vi "Title No. and Centroid.vi"(2 "半径":dbl, 3 "Particle Measurements (Pixels)":dbl[][](array[numeric])) -> (0 "粒子数":i32, 1 "输出数组":T1(array[cluster]))   [LabVIEW 2016]
panel:
  out "子数组":dbl[](array[numeric])
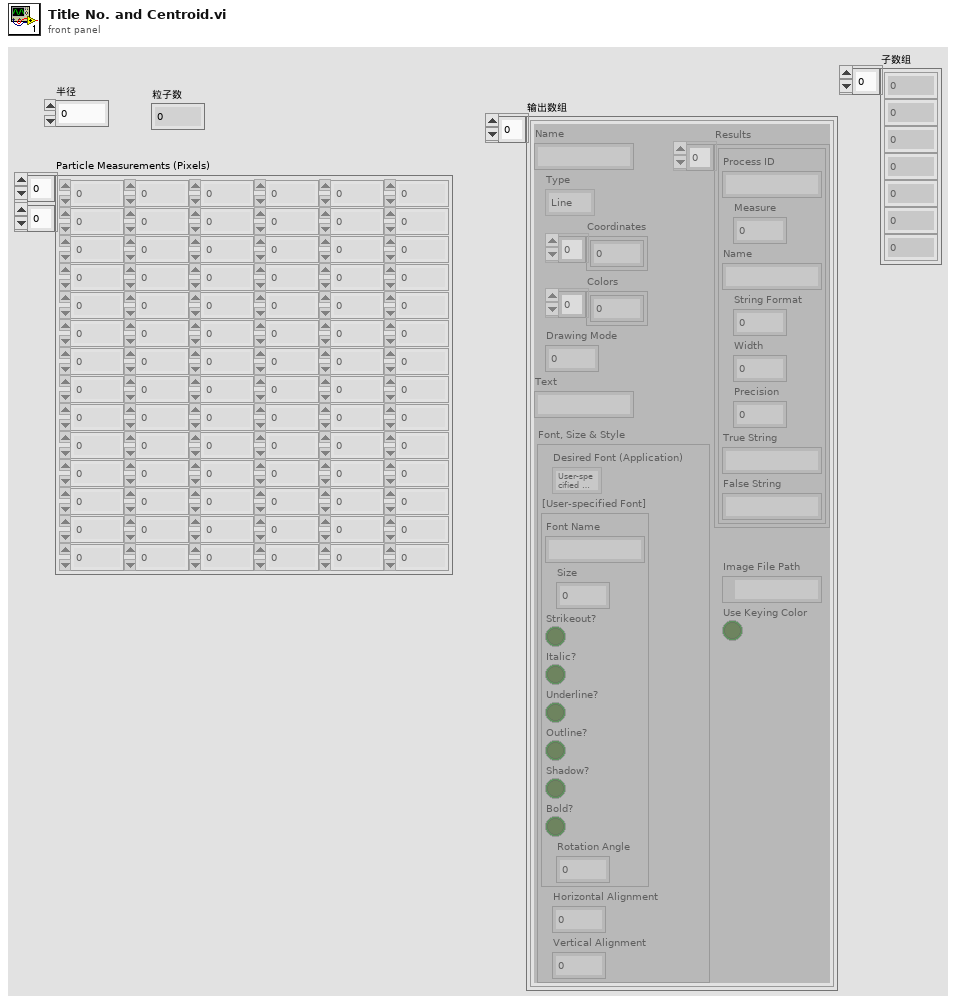
[diagram p1: front panel]
types:
  T1 = cluster{"Name":string, "Type":enum16{"Line", "Broken Line", "Free Hand Line", "Rotated Rectangle", "Oval", "Polygon", "Free Hand", "Bitmap", "Text"}, "Coordinates":i32[], "Colors":u32[], "Drawing Mode":u32, "Text":string, "Results":cluster{"Process ID":string, "Measure":u16, "Name":string, "String Format":u16, "Width":i16, "Precision":i16, "True String":string, "False String":string}[], "Font, Size & Style":cluster{"Desired Font (Application)":enum16{"User-specified Font", "Application Font", "System Font", "Dialog Font"}, "[User-specified Font]":cluster{"Font Name":string, "Size":i16, "Strikeout?":bool, "Italic?":bool, "Underline?":bool, "Outline?":bool, "Shadow?":bool, "Bold?":bool, "Rotation Angle":dbl}, "Horizontal Alignment":i16, "Vertical Alignment":i16}, "Image File Path":path, "Use Keying Color":bool}[]
  T2 = enum16{"Line", "Broken Line", "Free Hand Line", "Rotated Rectangle", "Oval", "Polygon", "Free Hand", "Bitmap", "Text"}
  T3 = cluster{"Name":string, "Type":enum16{"Line", "Broken Line", "Free Hand Line", "Rotated Rectangle", "Oval", "Polygon", "Free Hand", "Bitmap", "Text"}, "Coordinates":i32[], "Colors":u32[], "Drawing Mode":u32, "Text":string, "Results":cluster{"Process ID":string, "Measure":u16, "Name":string, "String Format":u16, "Width":i16, "Precision":i16, "True String":string, "False String":string}[], "Font, Size & Style":cluster{"Desired Font (Application)":enum16{"User-specified Font", "Application Font", "System Font", "Dialog Font"}, "[User-specified Font]":cluster{"Font Name":string, "Size":i16, "Strikeout?":bool, "Italic?":bool, "Underline?":bool, "Outline?":bool, "Shadow?":bool, "Bold?":bool, "Rotation Angle":dbl}, "Horizontal Alignment":i16, "Vertical Alignment":i16}, "Image File Path":path, "Use Keying Color":bool}
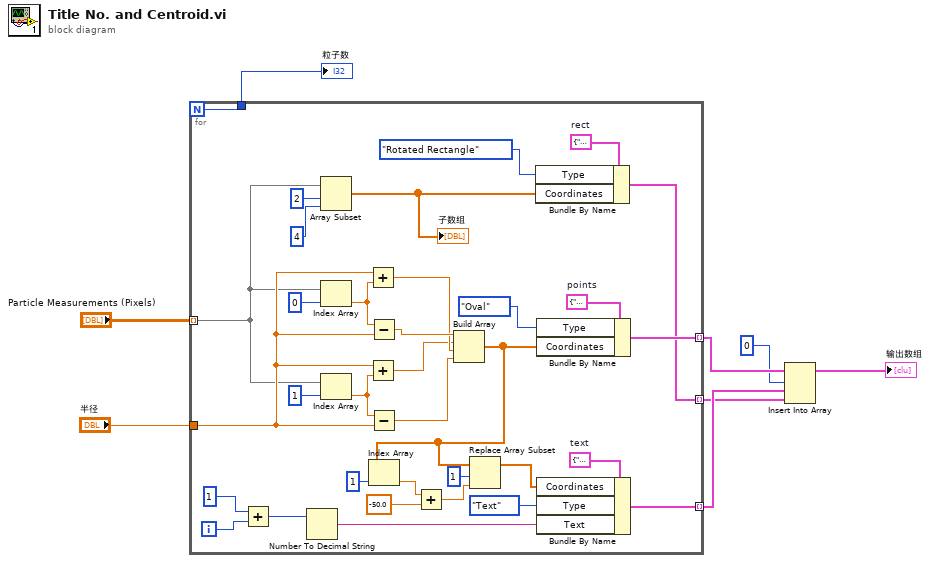
[diagram p0: block diagram]
diagram:
  n1 = for {
    N -> [w18]
    tunnel: "Particle Measurements (Pixels)" -> [w15] mode=indexing
    tunnel: "半径" -> [w38]
    tunnel: [w20] -> w6 mode=indexing
    tunnel: [w19] -> w5 mode=indexing
    tunnel: [w18] -> w2
    tunnel: [w11] -> w1 mode=indexing
    i -> [w25]
    w17 = T3 {"Name"="Oval 1", "Type"=enum."Oval", "Coordinates"=[1060, 662, 1162, 770], "Colors"=[3131392], "Drawing Mode"=0, "Text"="Your Text", "Results"=[], "Font, Size & Style"={"Desired Font (Application)"=enum."System Font", "[User-specified Font]"={"Font Name"="Tahoma", "Size"=13, "Strikeout?"=FALSE, "Italic?"=FALSE, "Underline?"=FALSE, "Outline?"=FALSE, "Shadow?"=FALSE, "Bold?"=FALSE, "Rotation Angle"=0.0}, "Horizontal Alignment"=0, "Vertical Alignment"=0}, "Image File Path"=path "", "Use Keying Color"=FALSE}  # rect
    w21 = T3 {"Name"="Oval 1", "Type"=enum."Oval", "Coordinates"=[1060, 662, 1162, 770], "Colors"=[3131392], "Drawing Mode"=1, "Text"="Your Text", "Results"=[], "Font, Size & Style"={"Desired Font (Application)"=enum."System Font", "[User-specified Font]"={"Font Name"="Tahoma", "Size"=13, "Strikeout?"=FALSE, "Italic?"=FALSE, "Underline?"=FALSE, "Outline?"=FALSE, "Shadow?"=FALSE, "Bold?"=FALSE, "Rotation Angle"=0.0}, "Horizontal Alignment"=0, "Vertical Alignment"=0}, "Image File Path"=path "", "Use Keying Color"=FALSE}  # points
    w22 = T3 {"Name"="Text 1", "Type"=enum."Text", "Coordinates"=[707, 439], "Colors"=[65280, 16777216], "Drawing Mode"=0, "Text"="Your Text", "Results"=[], "Font, Size & Style"={"Desired Font (Application)"=enum."System Font", "[User-specified Font]"={"Font Name"="Tahoma", "Size"=13, "Strikeout?"=FALSE, "Italic?"=FALSE, "Underline?"=FALSE, "Outline?"=FALSE, "Shadow?"=FALSE, "Bold?"=FALSE, "Rotation Angle"=0.0}, "Horizontal Alignment"=0, "Vertical Alignment"=0}, "Image File Path"=path "", "Use Keying Color"=FALSE}  # text
    n2 = Add(x=1, y=w25) -> (x+y=w23:i32)
    n3 = Number To Decimal String(number=w23) -> (decimal integer string=w33:string)  [unwired: 1 in]
    n4 = Array Subset(array=w15, index=2 ("索引"), length=4 ("长度")) -> (w12:dbl[])
    "子数组" <- w12
    n5 = Index Array(array=w15, index=0 ("索引")) -> (element=w41:dbl)
    n6 = Index Array(array=w15, index=1 ("索引")) -> (element=w40:dbl)
    n7 = Add(x=w38, y=w41) -> (x+y=w36:dbl)
    n8 = Add(x=w38, y=w40) -> (x+y=w10:dbl)
    n9 = Subtract(x=w41, y=w38) -> (x-y=w37:dbl)
    n10 = Subtract(x=w40, y=w38) -> (x-y=w9:dbl)
    n11 = Build Array(w37, w10, w36, w9) -> (w29:dbl[])
    n12 = Index Array(array=w29, index=1 ("索引")) -> (element=w31:dbl)
    n13 = Add(x=w31, y=-50.0) -> (x+y=w27:dbl)
    n14 = Replace Array Subset(array=w29, new element=w27, index=1 ("索引")) -> (w26:dbl[])
    n15 = Bundle By Name(cluster=w17, "Type"=T2."Rotated Rectangle", "Coordinates"=w12) -> (w11:T3)
    n16 = Bundle By Name(cluster=w21, "Type"=T2."Oval", "Coordinates"=w29) -> (w20:T3)
    n17 = Bundle By Name(cluster=w22, "Coordinates"=w26, "Type"=T2."Text", "Text"=w33) -> (w19:T3)
  }
  "粒子数" <- w2
  n18 = Insert Into Array(array=w6, index=0 ("索引"), new element #1=w5, new element #2=w1) -> (→"输出数组":T1)
